vi "GitHashToInfo.vi"(8 "error in (no error)":errorcluster, 9 "Directory":path=path "", 10 "Hash":string, 11 "Git exec":string="git") -> (0 "error out":errorcluster, 1 "Directory out":path, 2 "Commit Info":T1, 3 "Git exec out":string="git", 4 "Description":string)   [LabVIEW 2013]
uses:
  GitCommitCluster/CommitCluster.ctl
  GitCmd.vi
  <vilib>/dlg_ctls.llb/Space Constant.vi
  GitUtils/PathtoDirPath.vi
  <vilib>/Platform/system.llb/System Exec.vi
  <vilib>/Utility/error.llb/Error Cluster From Error Code.vi
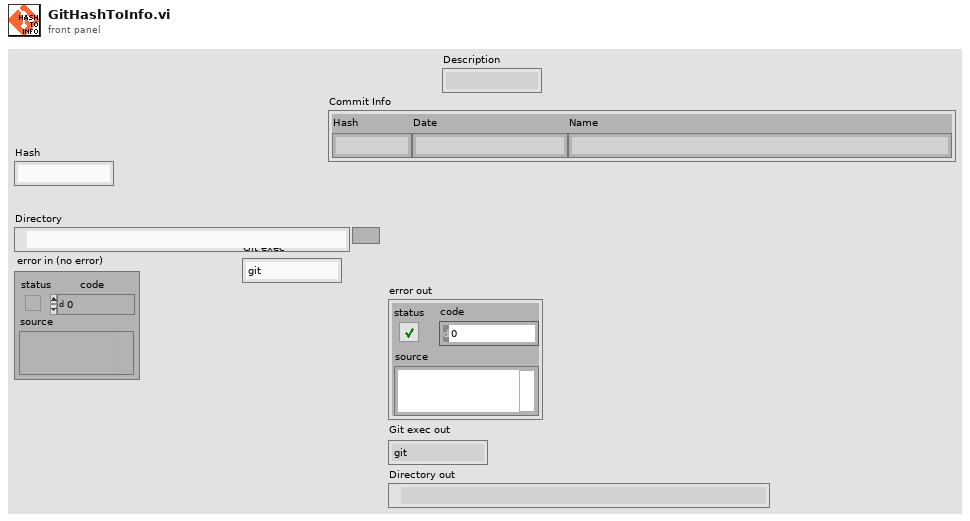
[diagram p1: front panel]
types:
  T1 = typedef "CommitCluster.ctl" = cluster{"Hash":string, "Date":string, "Name":string}
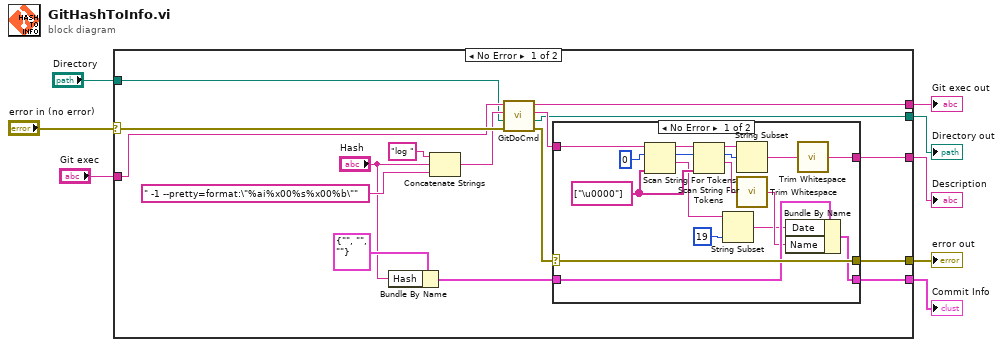
[diagram p0: block diagram]
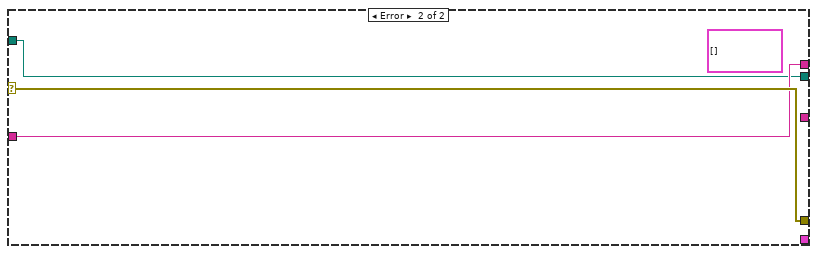
[diagram p3: hidden frame]
diagram:
  n1 = case shown="No Error" "error in (no error)" {
    selector: "error in (no error)" -> [w22 w46]
    tunnel: "Git exec" -> [w19 w45]
    tunnel: "Directory" -> [w15 w44]
    tunnel: [w23 w46] -> w6
    tunnel: [w18 w45] -> w4
    tunnel: [w16 w44] -> w3
    tunnel: [w13 _] -> w1
    tunnel: [w12 _] -> w2
    frame No Error {
      n2 = Bundle By Name(cluster=T1 {"Hash"="", "Date"="", "Name"=""} ("Commit"), "Hash"="Hash") -> (w10:T1)
      n3 = Concatenate Strings("log " ("string"), "Hash", " -1 --pretty=format:\"%ai%x00%s%x00%b\"" ("string")) -> (w20:string)
      n4 = call "GitDoCmd.vi"("error in (no error)"=w22, "Working Path"=w15, "Git command"=w20, "Git exec"=w19) -> ("error out"=w21:errorcluster, "Working Path out"=w16:path, "Returned stdout"=w17:string, "Git exec out"=w18:string)  [unwired: 3 in]
      n5 = case shown="No Error" w21 {
        selector: w21 -> [w41 w43]
        tunnel: w17 -> [w29 _]
        tunnel: [w41 w43] -> w23
        tunnel: [w34 w42] -> w13
        tunnel: [w36 _] -> w12
        tunnel: w10 -> [w35 w42]
        frame No Error {
          w32 = string[] ["\u0000"] ("delimiters (\\s,\\t,\\r,\\n)")
          n6 = Scan String For Tokens(6:w32, 8:0 ("offset"), 9:w29) -> (1:w25:string, 2:w31:i32, 3:w30:string)  [unwired: 3 in, 1 out]
          n7 = Scan String For Tokens(6:w32, 8:w31, 9:w30) -> (1:w37:string, 2:w39:i32, 3:w40:string)  [unwired: 3 in, 1 out]
          n8 = String Subset(string=w25, length (rest)=19 ("length (rest)")) -> (substring=w26:string)  [unwired: 1 in]
          n9 = String Subset(string=w40, offset (0)=w39) -> (substring=w38:string)  [unwired: 1 in]
          n10 = call <vilib>:"Trim Whitespace.vi"("string"=w37) -> ("trimmed string"=w33:string)  [unwired: 1 in]
          n11 = Bundle By Name(cluster=w35, "Date"=w26, "Name"=w33) -> (w34:T1)
          n12 = call <vilib>:"Trim Whitespace.vi"("string"=w38) -> ("trimmed string"=w36:string)  [unwired: 1 in]
        }
        frame Error {
        }
      }
    }
    frame Error {
      (unwired) T1[] [] ("Array")
    }
  }
  "error out" <- w6
  "Git exec out" <- w4
  "Directory out" <- w3
  "Description" <- w2
  "Commit Info" <- w1
